vi "omp.vi"(1 "N":i32, 2 "T":dbl[][](array[numeric]), 3 "s":dbl[](array[numeric])) -> (0 "hat_y":dbl[](array[numeric]))   [LabVIEW 2018]
uses:
  <vilib>/Analysis/_algsub.llb/Real Vector Norm.vi
  <vilib>/Analysis/baseanly.llb/Real Dot Product.vi
  <vilib>/Analysis/baseanly.llb/Real A x B.vi
  <vilib>/Analysis/baseanly.llb/A x Vector.vi
  <vilib>/Analysis/baseanly.llb/Real Inverse Matrix.vi
  <vilib>/Analysis/NI_AALBase.lvlib
  <vilib>/Analysis/NI_AALPro.lvlib
panel:
  out "r_n":dbl[](array[numeric])
  out "Aug_t":dbl[][](array[numeric])
  out "aug_y":dbl[](array[numeric]) format="%.2f"
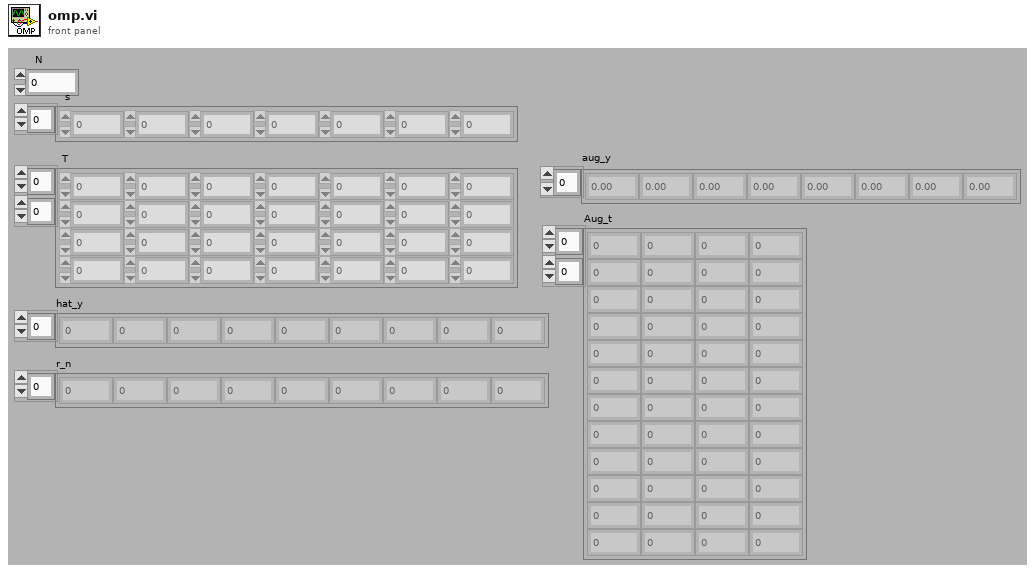
[diagram p1: front panel]
types:
  T1 = typedef "NI_Matrix.lvlib/RealMatrix.ctl" = dbl[][]
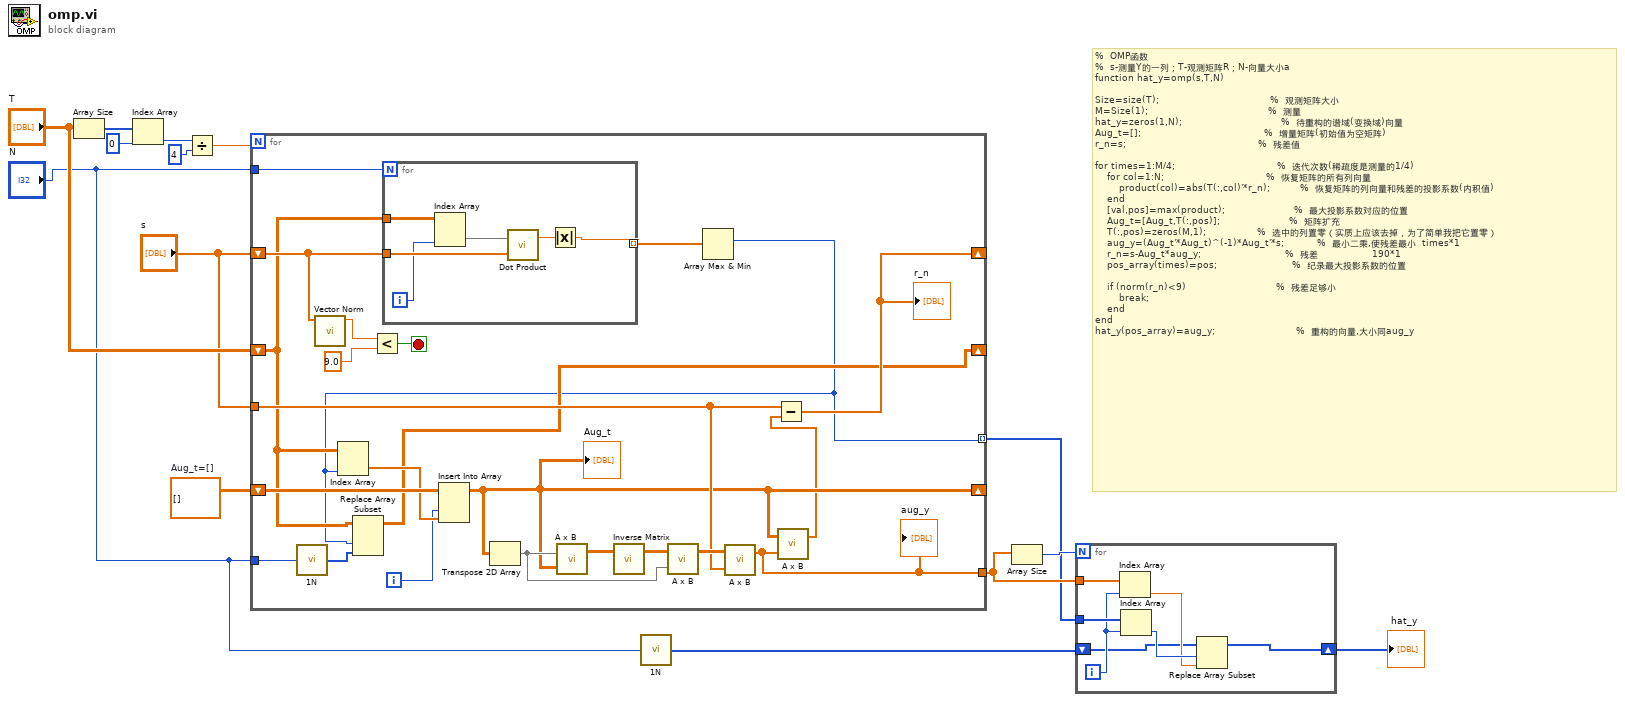
[diagram p0: block diagram]
diagram:
  w3 = dbl[][] []  # Aug_t=[]
  # "%  OMP函数\n%  s-测量Y的一列；T-观测矩阵R；N-向量大小a\nfunction hat_y=omp(s,T,N)\n\nSize=size(T);                                     %  观测矩阵大小\nM=Size(1);                                        %  测量\nhat_y=zeros(1,N);                                 %  待重构的谱域(变换域)向量\nAug_t=[];                                         %  增量矩阵(初始值为空矩阵)\nr_n=s;                                            %  残差值\n\nfor times=1:M/4;                                  %  迭代次数(稀疏度是测量的1/4)\n    for col=1:N;                                  %  恢复矩阵的所有列向量\n        product(col)=abs(T(:,col)'*r_n);          %  恢复矩阵的列向量和残差的投影系数(内积值) \n    end\n    [val,pos]=max(product);                       %  最大投影系数对应的位置\n    Aug_t=[Aug_t,T(:,pos)];                       %  矩阵扩充\n    T(:,pos)=zeros(M,1);                 %  选中的列置零（实质上应该去掉，为了简单我把它置零）\n    aug_y=(Aug_t'*Aug_t)^(-1)*Aug_t'*s;           %  最小二乘,使残差最小  times*1\n    r_n=s-Aug_t*aug_y;                            %  残差                  190*1\n    pos_array(times)=pos;                         %  纪录最大投影系数的位置\n    \n    if (norm(r_n)<9)                              %  残差足够小\n        break;\n    end\nend\nhat_y(pos_array)=aug_y;                           %  重构的向量,大小同aug_y"
  n1 = Array Size(array="T") -> (size(s)=w14:i32[])
  n2 = Index Array(array=w14, index=0 ("索引")) -> (element=w12:i32)
  n3 = Divide(x=w12, y=4) -> (x/y=w10:dbl)
  n4 = for {
    N: w10 -> [_]
    tunnel: "N" -> [w37]
    shift-right: [w30] -> _
    shift-left: "s" -> [w20]
    shift-right: [w24] -> _
    shift-left: w3 -> [w36]
    tunnel: "s" -> [w31]
    tunnel: [w26] -> w6
    shift-right: [w18] -> _
    shift-left: "T" -> [w19]
    tunnel: "N" -> [w23]
    tunnel: [w17] -> w2 mode=indexing
    i -> [w16]
    stop <- w27 stop-if-true
    n5 = call "1N.vi"("Numeric"=w23) -> ("Array"=w22:i32[])
    n6 = call-poly <vilib>:"Vector Norm.vi"("Input Vector"=w20) -> ("norm"=w29:dbl)  [unwired: 2 in, 8 out]
    n7 = Less?(x=w29, y=9.0) -> (x < y?=w27:bool)
    n8 = for {
      N: w37 -> [_]
      tunnel: w19 -> [w43]
      tunnel: w20 -> [w41]
      tunnel: [w38] -> w21 mode=indexing
      i -> [w39]
      n9 = Index Array(array=w43, index (col)=w39) -> (element=w42:dbl[])  [unwired: 1 in]
      n10 = call-poly <vilib>:"Dot Product.vi"("Y Vector"=w41, "X Vector"=w42) -> ("X * Y"=w40:dbl)  [unwired: 1 out]
      n11 = Absolute Value(x=w40) -> (abs(x)=w38:dbl)
    }
    n12 = Array Max & Min(array=w21) -> (max index (indices)=w17:i32)  [unwired: 3 out]
    n13 = Index Array(array=w19, index (col)=w17) -> (element=w35:dbl[])  [unwired: 1 in]
    n14 = Replace Array Subset(array=w19, new element=w22, index (col)=w17) -> (w18:dbl[][])  [unwired: 1 in]
    n15 = Insert Into Array "Insert Into Array"(array=w36, index (col)=w16, new element=w35) -> (w24:dbl[][])  [unwired: 1 in]
    "Aug_t" <- w24
    n16 = Transpose 2D Array(2D array=w24) -> (transposed array=w25:dbl[][])
    n17 = call-poly <vilib>:"A x B.vi"("B"=w24, "A"=w25) -> ("A x B"=w34:T1)  [unwired: 1 out]
    n18 = call-poly <vilib>:"Inverse Matrix.vi"("Input Matrix"=w34) -> ("Inverse Matrix"=w33:T1)  [unwired: 1 in, 1 out]
    n19 = call-poly <vilib>:"A x B.vi"("B"=w25, "A"=w33) -> ("A x B"=w32:T1)  [unwired: 1 out]
    n20 = call-poly <vilib>:"A x B.vi"("Vector"=w31, "A"=w32) -> ("A x Vector"=w26:dbl[])  [unwired: 1 out]
    "aug_y" <- w26
    n21 = call-poly <vilib>:"A x B.vi"("Vector"=w26, "A"=w24) -> ("A x Vector"=w15:dbl[])  [unwired: 1 out]
    n22 = Subtract(x=w31, y=w15) -> (x-y=w30:dbl[])
    "r_n" <- w30
  }
  n23 = call "1N.vi"("Numeric"="N") -> ("Array"=w4:i32[])
  n24 = Array Size(array=w6) -> (size(s)=w7:i32)
  n25 = for {
    N: w7 -> [_]
    tunnel: w6 -> [w50]
    tunnel: w2 -> [w49]
    shift-right: [w45] -> w5
    shift-left: w4 -> [w44]
    i -> [w48]
    n26 = Index Array(array=w50, index=w48) -> (element=w46:dbl)
    n27 = Index Array(array=w49, index=w48) -> (element=w47:i32)
    n28 = Replace Array Subset "Replace Array Subset"(array=w44, new element=w46, index=w47) -> (w45:i32[])
  }
  "hat_y" <- w5
